vi "produceTimingTicks.vi"(8 "error in (no error)":errorcluster, 10 "Channel":refnum<class "Channel.lvclass">, 11 "RampEvent in":refnum<class "RampEvent.lvclass">) -> (0 "error out":errorcluster, 2 "timingTickList":refnum<class "ScriptEventList.lvclass">, 3 "RampEvent out":refnum<class "RampEvent.lvclass">)   [LabVIEW 2009, in "Tools.lvlib" / "Scripting.lvlib" / "RampEvent.lvclass"]
uses:
  RampEvent.lvclass
  DatabaseHelpers/Database Objects/Channel/Channel.lvclass
  ScriptEventList/ScriptEventList.lvclass
  ScriptEvent.lvclass
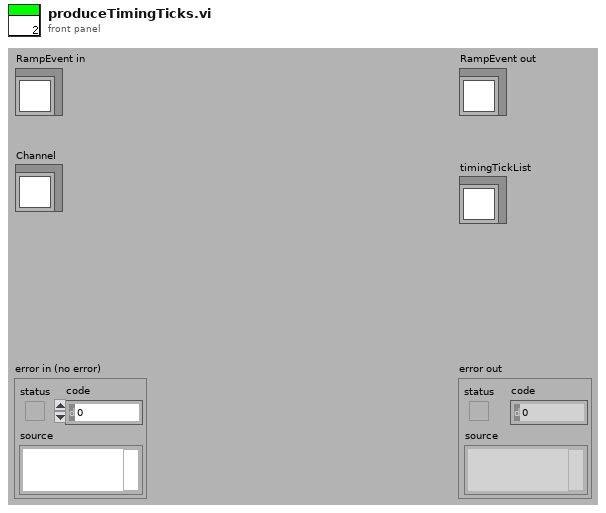
[diagram p1: front panel]
types:
  T1 = enum16{"changeValue", "pulse", "clock", "rampUp", "rampDown", "singleTone", "singleToneRamp", "playFile", "rf", "rfRamp"}
  T2 = enum16{"Initialise", "MOT", "Molasses", "Optical Pumping", "Magnetic Trap", "RF Cooling", "Manipulation", "Switch Off", "Absorption Imaging", "Fluorscence Imaging", "Shut Down"}
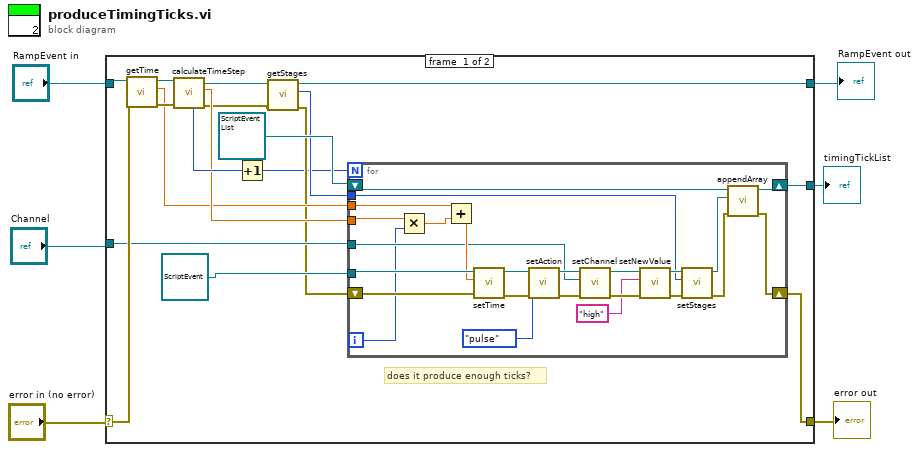
[diagram p0: block diagram]
diagram:
  n1 = case shown="No Error" "error in (no error)" {
    selector: "error in (no error)" -> [w20 w49]
    tunnel: "RampEvent in" -> [w21 w50]
    tunnel: [w16 w49] -> w2
    tunnel: [w8 w50] -> w4
    tunnel: "Channel" -> [w17 _]
    tunnel: [w14 _] -> w1
    frame #0 {
      # "does it produce enough ticks?"
      n2 = call "getTime.vi"("error in (no error)"=w20, "ScriptEvent.lvclass in"=w21) -> ("error out"=w19:errorcluster, "time"=w18:dbl, "ScriptEvent.lvclass out"=w22:refnum<class "RampEvent.lvclass">)  [unwired: 7 in]
      n3 = call "calculateTimeStep.vi"("error in (no error)"=w19, "RampEvent in"=w22) -> ("error out"=w11:errorcluster, "timeStep"=w23:dbl, "RampEvent out"=w12:refnum<class "RampEvent.lvclass">, "number of Steps"=w24:i32)  [unwired: 5 in, 1 out]
      n4 = Increment(x=w24) -> (x+1=w7:i32)
      n5 = call "getStages.vi"("error in (no error)"=w11, "ScriptEvent.lvclass in"=w12) -> ("error out"=w10:errorcluster, "Stage"=w9:T2, "ScriptEvent.lvclass out"=w8:refnum<class "RampEvent.lvclass">)  [unwired: 7 in]
      n6 = for {
        N: w7 -> [_]
        tunnel: w23 -> [w47]
        tunnel: w18 -> [w48]
        tunnel: refnum<class "ScriptEvent.lvclass"> refnum ("Tools.lvlib:Scripting.lvlib:ScriptEvent.lvclass") -> [w45]
        tunnel: w17 -> [w38]
        shift-right: [w31] -> w16
        shift-left: w10 -> [w43]
        shift-right: [w33] -> w14
        shift-left: refnum<class "ScriptEventList.lvclass"> refnum ("Tools.lvlib:Scripting.lvlib:ScriptEventList.lvclass") -> [w32]
        tunnel: w9 -> [w26]
        i -> [w34]
        n7 = Multiply(x=w47, y=w34) -> (x*y=w46:dbl)
        n8 = Add(x=w48, y=w46) -> (x+y=w44:dbl)
        n9 = call "setTime.vi"("error in (no error)"=w43, "time"=w44, "ScriptEvent.lvclass in"=w45) -> ("error out"=w41:errorcluster, "ScriptEvent.lvclass out"=w42:refnum<class "ScriptEvent.lvclass">)  [unwired: 7 in]
        n10 = call "setAction.vi"("error in (no error)"=w41, "action"=T1."pulse", "ScriptEvent.lvclass in"=w42) -> ("error out"=w39:errorcluster, "ScriptEvent.lvclass out"=w40:refnum<class "ScriptEvent.lvclass">)  [unwired: 7 in]
        n11 = call-dynamic "setChannel.vi"("error in (no error)"=w39, "Channel.lvclass"=w38, "ScriptEvent.lvclass in"=w40) -> ("error out"=w36:errorcluster, "ScriptEvent.lvclass out"=w37:refnum<class "ScriptEvent.lvclass">)  [unwired: 7 in]
        n12 = call "setNewValue.vi"("error in (no error)"=w36, "newValue"="high", "ScriptEvent.lvclass in"=w37) -> ("error out"=w29:errorcluster, "ScriptEvent.lvclass out"=w30:refnum<class "ScriptEvent.lvclass">)  [unwired: 7 in]
        n13 = call-dynamic "setStages.vi"("error in (no error)"=w29, "Stage"=w26, "ScriptEvent.lvclass in"=w30) -> ("error out"=w28:errorcluster, "ScriptEvent.lvclass out"=w27:refnum<class "ScriptEvent.lvclass">)  [unwired: 7 in]
        n14 = call "appendArray.vi"("error in (no error)"=w28, "ScriptEvent"=w27, "ScriptEventList in"=w32) -> ("error out"=w31:errorcluster, "ScriptEventList out"=w33:refnum<class "ScriptEventList.lvclass">)  [unwired: 6 in, 1 out]
      }
    }
    frame #1 {
    }
  }
  "error out" <- w2
  "RampEvent out" <- w4
  "timingTickList" <- w1
